vi "参数配置 (子VI).vi"(0 "温度":dbl, 1 "VISA resource name":refnum<visa-resource-name> caption="VISA资源名称", 4 "unit ID":u8=1 caption="单元ID", 12 "加标回收":dbl, 13 "硫酸":dbl, 14 "水样":dbl, 15 "蒸馏水":dbl, 16 "草酸钠":dbl, 17 "高锰酸钾":dbl, 18 "标液":dbl, 19 "质控样":dbl) -> ()   [LabVIEW 2016]
uses:
  <vilib>/Modbus/master/Create Master Instance (Serial).vi
  <vilib>/Modbus/master/Modbus Master.lvclass
panel:
  out "泵1计数":dbl
  out "泵2计数":dbl
  out "泵3计数":dbl
  out "泵4计数":dbl
  in  "标样浓度":dbl
  in  "标度泵计量数":dbl
  in  "零点泵计量数":dbl
  out "标度滴定值":dbl
  out "零点滴定值":dbl
  in  "关闭":bool
  in  "holding register values":u16[](array[numeric]) caption="保持寄存器值"
  in  "基本量程":enum16{"10mL", "20mL"}(ring)
  in  "修正系数":dbl
  in  "浓度":dbl
  in  "恒温时间":dbl
  # "基本参数设置"
  # "泵计量参数设置"
  # "校零校标结果"
  # "水样："
  # "高锰酸钾："
  # "校零结果："
  # "校零滴定值："
  # "零点泵计量值："
  # "加热恒温温度（℃）："
  # "校标结果："
  # "标度滴定值："
  # "恒温时间（分钟）："
  # "蒸馏水："
  # "草酸钠："
  # "标度泵计量值："
  # "标样浓度："
  # "标准液浓度（mg/L）："
  # "标液："
  # "硫酸："
  # "质控样："
  # "修正系数："
  # "加标回收样："
  # "基本量程（20mL可选）："
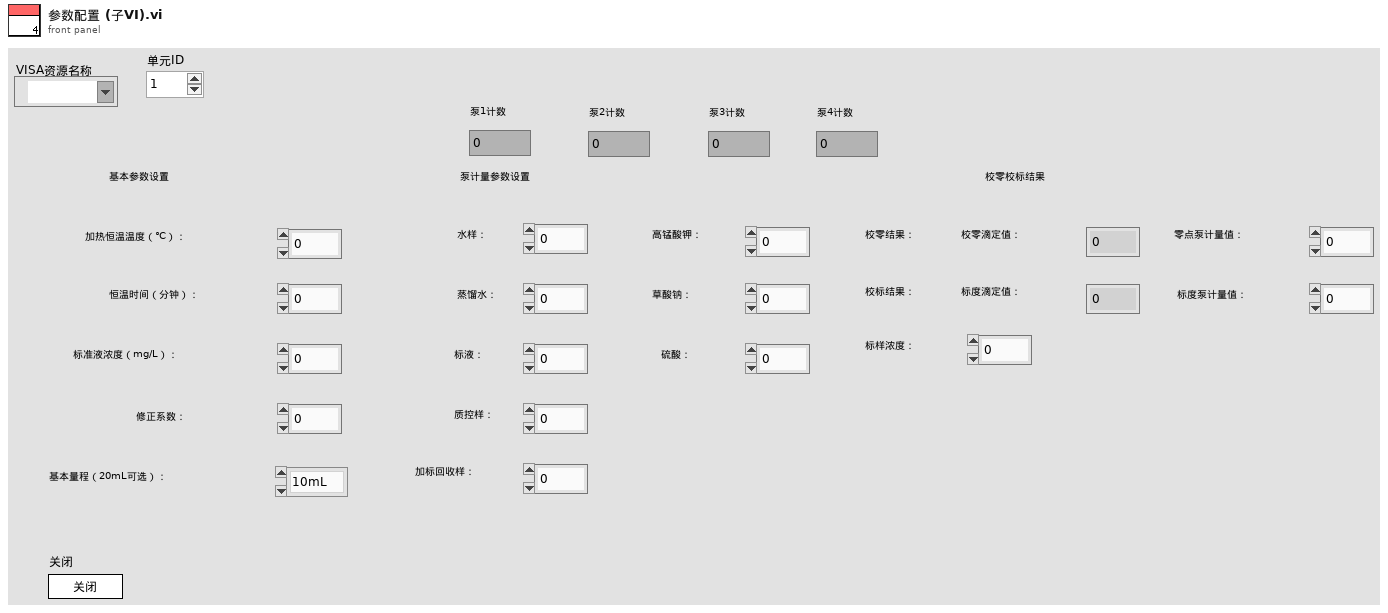
[diagram p1: front panel]
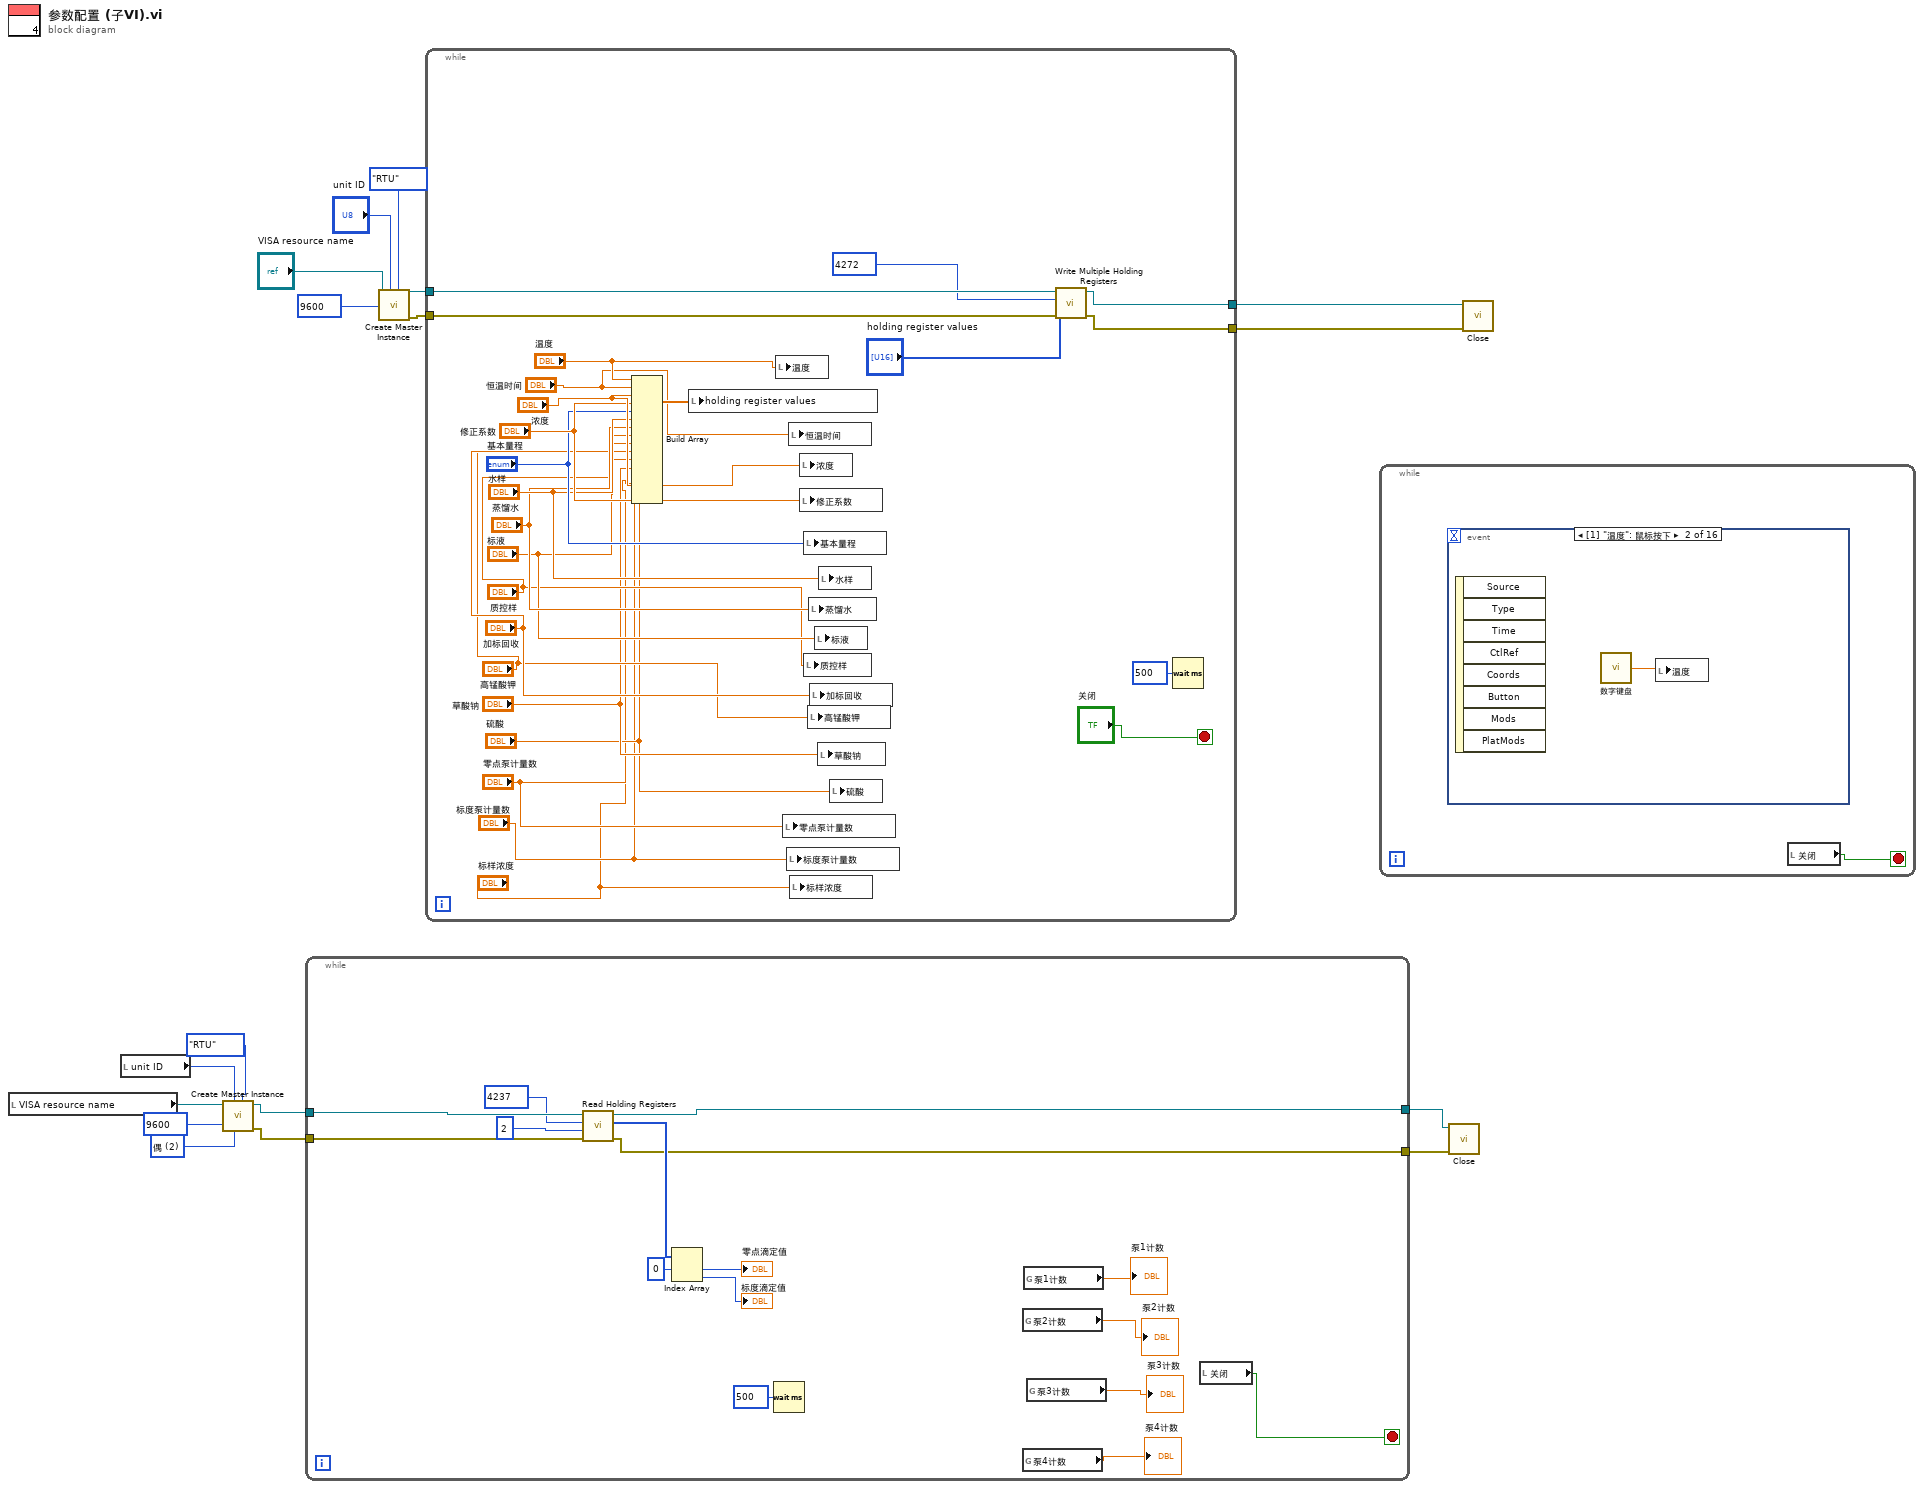
[diagram p0: block diagram]
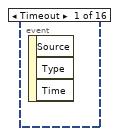
[diagram p2: hidden frame]
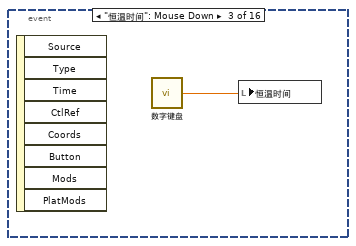
[diagram p3: hidden frame]
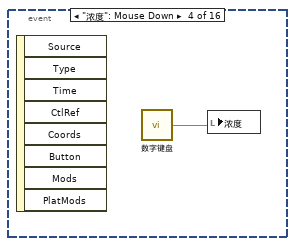
[diagram p4: hidden frame]
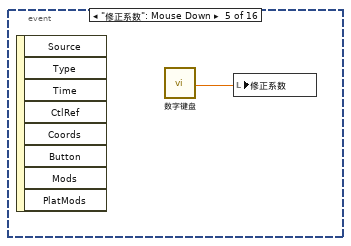
[diagram p5: hidden frame]
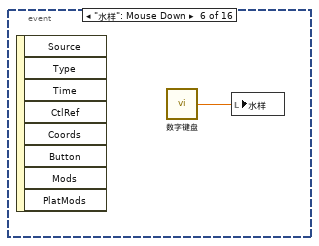
[diagram p6: hidden frame]
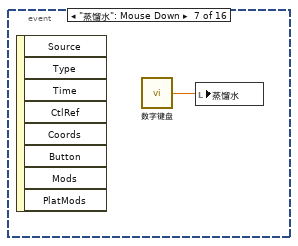
[diagram p7: hidden frame]
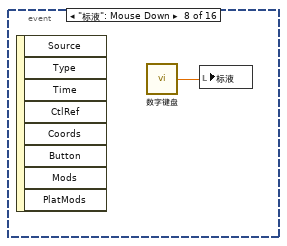
[diagram p8: hidden frame]
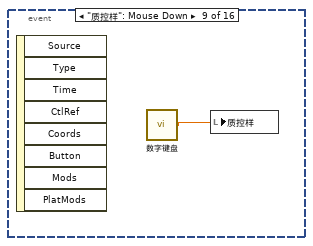
[diagram p9: hidden frame]
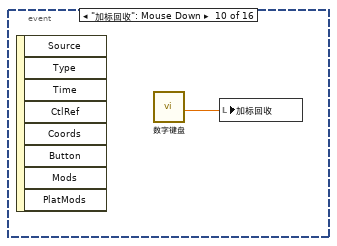
[diagram p10: hidden frame]
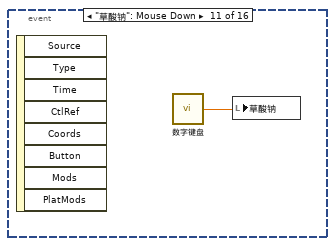
[diagram p11: hidden frame]
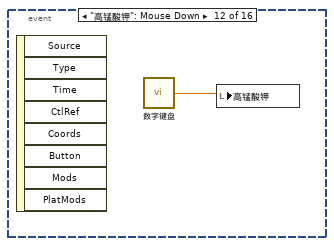
[diagram p12: hidden frame]
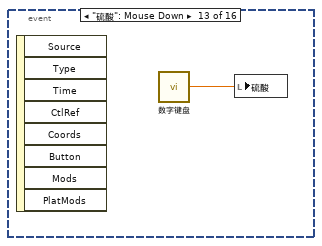
[diagram p13: hidden frame]
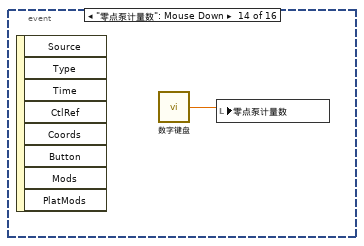
[diagram p14: hidden frame]
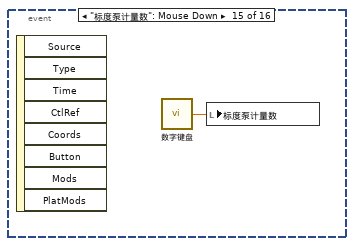
[diagram p15: hidden frame]
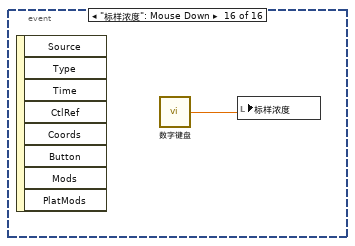
[diagram p16: hidden frame]
diagram:
  w1 = u16 2 items=["无", "奇", "偶"] ("parity (Even)")
  n1 = local read "VISA resource name"() -> (w7:refnum<visa-resource-name>)
  n2 = local read "unit ID"() -> (w8:u8)
  n3 = call-poly <vilib>:"Create Master Instance.vi"("serial type"=enum16{"RTU", "ASCII"}."RTU", "parity (Even)"=w1, "unit ID"=w8, "baud rate (9600)"=u32 9600, "VISA resource name"=w7) -> ("error out"=w5:errorcluster, "serial master instance"=w6:refnum<class "Modbus Master.lvclass">)  [unwired: 5 in]
  n4 = while {
    tunnel: w6 -> [w27]
    tunnel: w5 -> [w26]
    tunnel: [w19] -> w4
    tunnel: [w18] -> w3
    stop <- w32 stop-if-true
    n5 = call-dynamic "Read Holding Registers.vi"("error in (no error)"=w26, "number of holding registers"=u16 2, "starting address"=u16 4237, "Modbus master in"=w27) -> ("error out"=w18:errorcluster, "register values"=w23:u16[], "Modbus master out"=w19:refnum<class "Modbus Master.lvclass">)  [unwired: 5 in]
    n6 = Index Array(array=w23, index #1=0 ("索引")) -> (element #1=→"零点滴定值":u16, element #2=→"标度滴定值":u16)  [unwired: 1 in]
    n7 = Wait (ms)(milliseconds to wait=u32 500 ("等待时间（毫秒）")) -> ()  [unwired: 1 out]
    n8 = global read "泵计数全局.vi" "泵2计数"() -> (→"泵2计数":dbl)
    n9 = global read "泵计数全局.vi" "泵4计数"() -> (→"泵4计数":dbl)
    n10 = global read "泵计数全局.vi" "泵1计数"() -> (→"泵1计数":dbl)
    n11 = global read "泵计数全局.vi" "泵3计数"() -> (→"泵3计数":dbl)
    n12 = local read "关闭"() -> (w32:bool)
  }
  n13 = call-poly <vilib>:"Create Master Instance.vi"("serial type"=enum16{"RTU", "ASCII"}."RTU", "unit ID"="unit ID", "baud rate (9600)"=u32 9600, "VISA resource name"="VISA resource name") -> ("error out"=w12:errorcluster, "serial master instance"=w17:refnum<class "Modbus Master.lvclass">)  [unwired: 6 in]
  n14 = while {
    tunnel: w17 -> [w58]
    tunnel: w12 -> [w57]
    tunnel: [w54] -> w11
    tunnel: [w53] -> w10
    stop <- "关闭" stop-if-true
    n15 = Build Array("温度", "恒温时间", "浓度", "修正系数", "基本量程", "水样", "蒸馏水", "标液", "质控样", "加标回收", "高锰酸钾", "草酸钠", "硫酸", "零点泵计量数", "标度泵计量数", "标样浓度") -> (w52:dbl[])
    n16 = local write "holding register values"(w52) -> ()
    n17 = local write "温度"("温度") -> ()
    n18 = local write "零点泵计量数"("零点泵计量数") -> ()
    n19 = local write "标度泵计量数"("标度泵计量数") -> ()
    n20 = local write "恒温时间"("恒温时间") -> ()
    n21 = local write "标样浓度"("标样浓度") -> ()
    n22 = local write "浓度"("浓度") -> ()
    n23 = local write "修正系数"("修正系数") -> ()
    n24 = local write "基本量程"("基本量程") -> ()
    n25 = local write "质控样"("质控样") -> ()
    n26 = local write "高锰酸钾"("高锰酸钾") -> ()
    n27 = local write "蒸馏水"("蒸馏水") -> ()
    n28 = local write "加标回收"("加标回收") -> ()
    n29 = local write "标液"("标液") -> ()
    n30 = local write "草酸钠"("草酸钠") -> ()
    n31 = local write "水样"("水样") -> ()
    n32 = local write "硫酸"("硫酸") -> ()
    n33 = call-dynamic "Write Multiple Holding Registers.vi"("error in (no error)"=w57, "holding register values"="holding register values", "starting address"=u16 4272, "Modbus master in"=w58) -> ("error out"=w53:errorcluster, "Modbus master out"=w54:refnum<class "Modbus Master.lvclass">)  [unwired: 6 in]
    n34 = Wait (ms)(milliseconds to wait=u32 500 ("等待时间（毫秒）")) -> ()  [unwired: 1 out]
  }
  n35 = while {
    stop <- w59 stop-if-true
    n36 = event shown="[1] \"温度\": 鼠标按下" {
      selector: _ -> [_ _ _ _ _ _ _ _ _ _ _ _ _ _ _ _]
      dyn-events: _ -> [_ _ _ _ _ _ _ _ _ _ _ _ _ _ _ _]
      timeout: _ -> [_ _ _ _ _ _ _ _ _ _ _ _ _ _ _ _]
      event Timeout {
        n37 = event-data() -> ()  [unwired: 1 in, 3 out]
      }
      event "温度": Mouse Down {
        n38 = event-data() -> ()  [unwired: 1 in, 8 out]
        n39 = call "数字键盘.vi"() -> ("NewNumber"=w60:sgl)  [unwired: 1 in]
        n40 = local write "温度"(w60) -> ()
      }
      event "恒温时间": Mouse Down {
        n41 = event-data() -> ()  [unwired: 1 in, 8 out]
        n42 = call "数字键盘.vi"() -> ("NewNumber"=w61:sgl)  [unwired: 1 in]
        n43 = local write "恒温时间"(w61) -> ()
      }
      event "浓度": Mouse Down {
        n44 = event-data() -> ()  [unwired: 1 in, 8 out]
        n45 = call "数字键盘.vi"() -> ("NewNumber"=w62:sgl)  [unwired: 1 in]
        n46 = local write "浓度"(w62) -> ()
      }
      event "修正系数": Mouse Down {
        n47 = event-data() -> ()  [unwired: 1 in, 8 out]
        n48 = call "数字键盘.vi"() -> ("NewNumber"=w63:sgl)  [unwired: 1 in]
        n49 = local write "修正系数"(w63) -> ()
      }
      event "水样": Mouse Down {
        n50 = event-data() -> ()  [unwired: 1 in, 8 out]
        n51 = call "数字键盘.vi"() -> ("NewNumber"=w64:sgl)  [unwired: 1 in]
        n52 = local write "水样"(w64) -> ()
      }
      event "蒸馏水": Mouse Down {
        n53 = event-data() -> ()  [unwired: 1 in, 8 out]
        n54 = call "数字键盘.vi"() -> ("NewNumber"=w65:sgl)  [unwired: 1 in]
        n55 = local write "蒸馏水"(w65) -> ()
      }
      event "标液": Mouse Down {
        n56 = event-data() -> ()  [unwired: 1 in, 8 out]
        n57 = call "数字键盘.vi"() -> ("NewNumber"=w66:sgl)  [unwired: 1 in]
        n58 = local write "标液"(w66) -> ()
      }
      event "质控样": Mouse Down {
        n59 = event-data() -> ()  [unwired: 1 in, 8 out]
        n60 = call "数字键盘.vi"() -> ("NewNumber"=w67:sgl)  [unwired: 1 in]
        n61 = local write "质控样"(w67) -> ()
      }
      event "加标回收": Mouse Down {
        n62 = event-data() -> ()  [unwired: 1 in, 8 out]
        n63 = call "数字键盘.vi"() -> ("NewNumber"=w68:sgl)  [unwired: 1 in]
        n64 = local write "加标回收"(w68) -> ()
      }
      event "草酸钠": Mouse Down {
        n65 = event-data() -> ()  [unwired: 1 in, 8 out]
        n66 = call "数字键盘.vi"() -> ("NewNumber"=w69:sgl)  [unwired: 1 in]
        n67 = local write "草酸钠"(w69) -> ()
      }
      event "高锰酸钾": Mouse Down {
        n68 = event-data() -> ()  [unwired: 1 in, 8 out]
        n69 = call "数字键盘.vi"() -> ("NewNumber"=w70:sgl)  [unwired: 1 in]
        n70 = local write "高锰酸钾"(w70) -> ()
      }
      event "硫酸": Mouse Down {
        n71 = event-data() -> ()  [unwired: 1 in, 8 out]
        n72 = call "数字键盘.vi"() -> ("NewNumber"=w71:sgl)  [unwired: 1 in]
        n73 = local write "硫酸"(w71) -> ()
      }
      event "零点泵计量数": Mouse Down {
        n74 = event-data() -> ()  [unwired: 1 in, 8 out]
        n75 = call "数字键盘.vi"() -> ("NewNumber"=w72:sgl)  [unwired: 1 in]
        n76 = local write "零点泵计量数"(w72) -> ()
      }
      event "标度泵计量数": Mouse Down {
        n77 = event-data() -> ()  [unwired: 1 in, 8 out]
        n78 = call "数字键盘.vi"() -> ("NewNumber"=w73:sgl)  [unwired: 1 in]
        n79 = local write "标度泵计量数"(w73) -> ()
      }
      event "标样浓度": Mouse Down {
        n80 = event-data() -> ()  [unwired: 1 in, 8 out]
        n81 = call "数字键盘.vi"() -> ("NewNumber"=w74:sgl)  [unwired: 1 in]
        n82 = local write "标样浓度"(w74) -> ()
      }
    }
    n83 = local read "关闭"() -> (w59:bool)
  }
  n84 = call-dynamic "Close.vi"("error in (no error)"=w3, "Modbus master in"=w4) -> ()  [unwired: 9 in, 1 out]
  n85 = call-dynamic "Close.vi"("error in (no error)"=w10, "Modbus master in"=w11) -> ()  [unwired: 9 in, 1 out]
